vi "AddBatchRuns_DP_ver1.0.vi"(1 "output cluster":T1={"Main Sweep"=0, "Steps Config:"={"total points:"=0, "Step Delay (s)"=0.0, "Ini Delay (s)"=0.0, "# of steps:"=0}, "Temperature Control (ITC 503):"={"GPIB ADR"=0, "Change Heater?"={"Heater?"=FALSE, "Heater"=0}, "Change Temp?"={"Change T?"=FALSE, "Set T (K)"=0.0}, "Cluster"={"Heat Auto?"=FALSE, "Manual Heat?"=FALSE, "Heater (%)"=0.0}, "Change PID?"={"Change PID?"=FALSE, "P"=0.0, "I"=0.0, "D"=0.0}, "Change Para?"=FALSE, "Sensor"=1}, "Temperature Control (LS 340):"={"GPIB ADR"=0, "From (K)"=0.0, "To (K)"=0.0, "Rate (K/min)"=0.0, "Delta T (0.08K)"=0.0, "Temp. Header"="", "T Display Control"={"Ch B"=FALSE, "Ch C"=FALSE, "Ch D"=FALSE}}, "Magnet Control (IPS 120-10)"={"Action"=0, "Standby (s)"=0.0, "Heater on (s)"=0.0, "Sweep Setup "=[], "GPIB ADR"=0, "Change Para?"=FALSE}, "Keithley 6221 :"=[], "Measuring Instruments : "=[], "Lock-In SR7265 :"=[], "Deascription of \nthis measurement"="", "Instruments Config:"=[], "LS372 Bridge : 2"=[{"GPIB"=0, "Excitation"=0, "Autorange?"=FALSE, "Range"=0, "Current"=0, "Voltage"=0, "DataHeader"="Rx;Ry"}], "Magnet Control (CS4) 2"={"Action"=1, "Standby (s)"=0.0, "Heater on (s)"=300.0, "Sweep Setup "=[], "GPIB ADR"=0, "Change Para?"=FALSE}} {"Magnet Control (CS4) 2"."GPIB ADR" items=["None"=0, "25"=25]; "Magnet Control (CS4) 2"."Sweep Setup"."Rate in Range (T/min)" min=0.001 max=0.5 step=0.001; "Magnet Control (CS4) 2"."Sweep Setup"."Hold(min)" min=0.0; "Magnet Control (CS4) 2"."Sweep Setup"."Set Point (T)" min=-9.0 max=9.0 step=0.001; "Magnet Control (CS4) 2"."Action" items=["Up", "Down", "Pause", "Zero"]; "LS372 Bridge : 2"."Voltage" items=["2.00 uV"=1, "6.32 uV"=2, "20.0 uV"=3, "63.2 uV"=4, "200 uV"=5, "632 uV"=6, "2.0 mV"=7, "6.32 mV"=8]; "LS372 Bridge : 2"."Current" items=["1.00 pA"=1, "3.16 pA"=2, "10.0 pA"=3, "31.6 pA"=4, "100 pA"=5, "316 pA"=6, "1.00 nA"=7, "3.16 nA"=8, "10 nA"=9, "31.6 nA"=10, "100 nA"=11, "316 nA"=12, "1.00 uA"=13, "3.16 uA"=14, "10.0 uA"=15, "31.6 uA"=16, "100 uA"=17, "316 uA"=18, "1.00 mA"=19, "3.16 mA"=20, "10.0 mA"=21, "31.6 mA"=22]; "LS372 Bridge : 2"."Range" items=["2.0 m"=1, "6.32 m"=2, "20.0 m"=3, "63.2 m"=4, "200 m"=5, "632 m"=6, "2.00"=7, "6.32"=8, "20.0"=9, "63.2"=10, "200"=11, "632"=12, "2.00 k"=13, "6.32 k"=14, "20.0 k"=15, "63.2 k"=16, "200 k"=17, "632 k"=18, "2.00 M"=19, "6.32 M"=20, "20.0 M"=21, "63.2 M"=22]; "LS372 Bridge : 2"."Excitation" items=["Voltage", "Current"]; "LS372 Bridge : 2"."GPIB" items=["None"=0, "9"=9]; "Main Sweep" items=["Time", "DC Current", "Delta Current", "Pulse Delta Current", "Sine Current", "Lock-in Vosc"]; "Temperature Control (ITC 503):"."Sensor" items=["T2", "T3"]; "Magnet Control (IPS 120-10)"."Action" items=["Hold", "To Set point", "To Zero", "Clamp"]; "Keithley 6221 :"."Sweep Mode" items=["Linear", "Log", "Exp", "Inverse", "Manual"]}) -> (0 "output cluster 2":T1={"Main Sweep"=0, "Steps Config:"={"total points:"=0, "Step Delay (s)"=0.0, "Ini Delay (s)"=0.0, "# of steps:"=0}, "Temperature Control (ITC 503):"={"GPIB ADR"=0, "Change Heater?"={"Heater?"=FALSE, "Heater"=0}, "Change Temp?"={"Change T?"=FALSE, "Set T (K)"=0.0}, "Cluster"={"Heat Auto?"=FALSE, "Manual Heat?"=FALSE, "Heater (%)"=0.0}, "Change PID?"={"Change PID?"=FALSE, "P"=0.0, "I"=0.0, "D"=0.0}, "Change Para?"=FALSE, "Sensor"=1}, "Temperature Control (LS 340):"={"GPIB ADR"=0, "From (K)"=0.0, "To (K)"=0.0, "Rate (K/min)"=0.0, "Delta T (0.08K)"=0.0, "Temp. Header"="", "T Display Control"={"Ch B"=FALSE, "Ch C"=FALSE, "Ch D"=FALSE}}, "Magnet Control (IPS 120-10)"={"Action"=0, "Standby (s)"=0.0, "Heater on (s)"=0.0, "Sweep Setup "=[], "GPIB ADR"=0, "Change Para?"=FALSE}, "Keithley 6221 :"=[], "Measuring Instruments : "=[], "Lock-In SR7265 :"=[], "Deascription of \nthis measurement"="", "Instruments Config:"=[], "LS372 Bridge : 2"=[{"GPIB"=0, "Excitation"=0, "Autorange?"=FALSE, "Range"=0, "Current"=0, "Voltage"=0, "DataHeader"="Rx;Ry"}], "Magnet Control (CS4) 2"={"Action"=1, "Standby (s)"=0.0, "Heater on (s)"=300.0, "Sweep Setup "=[], "GPIB ADR"=0, "Change Para?"=FALSE}} {"Magnet Control (CS4) 2"."GPIB ADR" items=["None"=0, "25"=25]; "Magnet Control (CS4) 2"."Sweep Setup"."Rate in Range (T/min)" min=0.001 max=0.5 step=0.001; "Magnet Control (CS4) 2"."Sweep Setup"."Hold(min)" min=0.0; "Magnet Control (CS4) 2"."Sweep Setup"."Set Point (T)" min=-9.0 max=9.0 step=0.001; "Magnet Control (CS4) 2"."Action" items=["Up", "Down", "Pause", "Zero"]; "LS372 Bridge : 2"."Voltage" items=["2.00 uV"=1, "6.32 uV"=2, "20.0 uV"=3, "63.2 uV"=4, "200 uV"=5, "632 uV"=6, "2.0 mV"=7, "6.32 mV"=8]; "LS372 Bridge : 2"."Current" items=["1.00 pA"=1, "3.16 pA"=2, "10.0 pA"=3, "31.6 pA"=4, "100 pA"=5, "316 pA"=6, "1.00 nA"=7, "3.16 nA"=8, "10 nA"=9, "31.6 nA"=10, "100 nA"=11, "316 nA"=12, "1.00 uA"=13, "3.16 uA"=14, "10.0 uA"=15, "31.6 uA"=16, "100 uA"=17, "316 uA"=18, "1.00 mA"=19, "3.16 mA"=20, "10.0 mA"=21, "31.6 mA"=22]; "LS372 Bridge : 2"."Range" items=["2.0 m"=1, "6.32 m"=2, "20.0 m"=3, "63.2 m"=4, "200 m"=5, "632 m"=6, "2.00"=7, "6.32"=8, "20.0"=9, "63.2"=10, "200"=11, "632"=12, "2.00 k"=13, "6.32 k"=14, "20.0 k"=15, "63.2 k"=16, "200 k"=17, "632 k"=18, "2.00 M"=19, "6.32 M"=20, "20.0 M"=21, "63.2 M"=22]; "LS372 Bridge : 2"."Excitation" items=["Voltage", "Current"]; "LS372 Bridge : 2"."GPIB" items=["None"=0, "9"=9]; "Main Sweep" items=["Time", "DC Current", "Delta Current", "Pulse Delta Current", "Sine Current", "Lock-in Vosc"]; "Temperature Control (ITC 503):"."Sensor" items=["T2", "T3"]; "Magnet Control (IPS 120-10)"."Action" items=["Hold", "To Set point", "To Zero", "Clamp"]; "Keithley 6221 :"."Sweep Mode" items=["Linear", "Log", "Exp", "Inverse", "Manual"]})   [LabVIEW 2012]
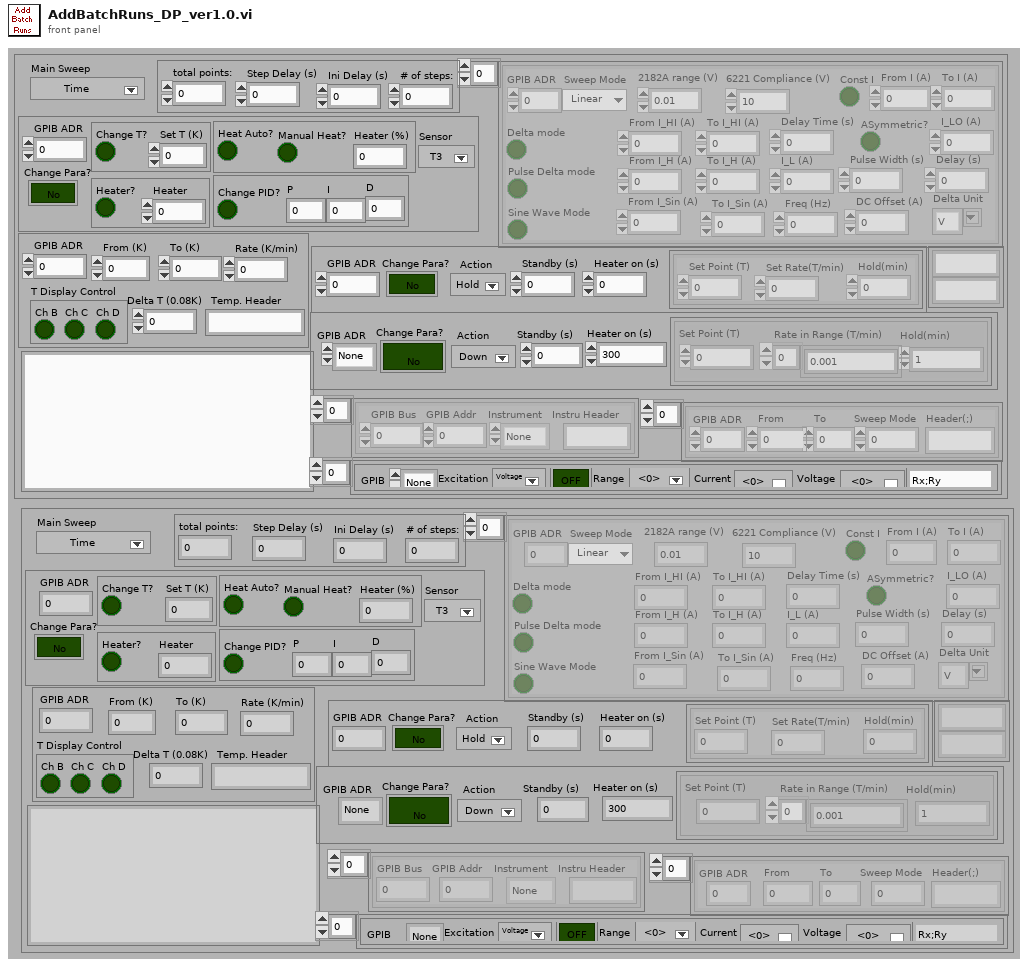
[diagram p1: front panel]
types:
  T1 = cluster{"Main Sweep":u8, "Steps Config:":cluster{"total points:":u32, "Step Delay (s)":dbl, "Ini Delay (s)":dbl, "# of steps:":u32}, "Temperature Control (ITC 503):":cluster{"GPIB ADR":u16, "Change Heater?":cluster{"Heater?":bool, "Heater":u8}, "Change Temp?":cluster{"Change T?":bool, "Set T (K)":dbl}, "Cluster":cluster{"Heat Auto?":bool, "Manual Heat?":bool, "Heater (%)":dbl}, "Change PID?":cluster{"Change PID?":bool, "P":dbl, "I":dbl, "D":dbl}, "Change Para?":bool, "Sensor":u16}, "Temperature Control (LS 340):":cluster{"GPIB ADR":u16, "From (K)":dbl, "To (K)":dbl, "Rate (K/min)":dbl, "Delta T (0.08K)":dbl, "Temp. Header":string, "T Display Control":cluster{"Ch B":bool, "Ch C":bool, "Ch D":bool}}, "Magnet Control (IPS 120-10)":cluster{"Action":u16, "Standby (s)":dbl, "Heater on (s)":dbl, "Sweep Setup ":cluster{"Set Point (T)":dbl, "Set Rate(T/min)":dbl, "Hold(min)":dbl}[], "GPIB ADR":u16, "Change Para?":bool}, "Keithley 6221 :":cluster{"Delta mode":bool, "Const I":bool, "Pulse Delta mode":bool, "Sine Wave Mode":bool, "From I_HI (A)":dbl, "From I (A)":dbl, "I_LO (A)":dbl, "From I_H (A)":dbl, "I_L (A)":dbl, "Freq (Hz)":dbl, "From I_Sin (A)":dbl, "DC Offset (A)":dbl, "Delay Time (s)":dbl, "Pulse Width (s)":dbl, "Delay (s)":dbl, "To I (A)":dbl, "ASymmetric?":bool, "To I_HI (A)":dbl, "To I_H (A)":dbl, "To I_Sin (A)":dbl, "GPIB ADR":u16, "Sweep Mode":u8, "Delta Unit":string, "2182A range (V)":dbl, "6221 Compliance (V)":dbl}[], "Measuring Instruments : ":cluster{"GPIB Bus":dbl, "GPIB Addr":dbl, "Instrument":enum16{"None", "HP34401DMM", "Lockin 7265", "HP3456/7A", "HP3478A", "HP3325FG", "Keithley2182A"}, "Instru Header":string}[], "Lock-In SR7265 :":cluster{"GPIB ADR":u16, "From":dbl, "To":dbl, "Header(;)":string, "Sweep Mode":u8}[], "Deascription of \nthis measurement":string, "Instruments Config:":string[][], "LS372 Bridge : 2":cluster{"GPIB":u16, "Excitation":u16, "Autorange?":bool, "Range":u16, "Current":u16, "Voltage":u16, "DataHeader":string}[], "Magnet Control (CS4) 2":cluster{"Action":u16, "Standby (s)":dbl, "Heater on (s)":dbl, "Sweep Setup ":cluster{"Set Point (T)":dbl, "Hold(min)":dbl, "Rate in Range (T/min)":dbl[]}[], "GPIB ADR":u16, "Change Para?":bool}}
  T2 = cluster{"Delta mode":bool, "Const I":bool, "Pulse Delta mode":bool, "Sine Wave Mode":bool, "From I_HI (A)":dbl, "From I (A)":dbl, "I_LO (A)":dbl, "From I_H (A)":dbl, "I_L (A)":dbl, "Freq (Hz)":dbl, "From I_Sin (A)":dbl, "DC Offset (A)":dbl, "Delay Time (s)":dbl, "Pulse Width (s)":dbl, "Delay (s)":dbl, "To I (A)":dbl, "ASymmetric?":bool, "To I_HI (A)":dbl, "To I_H (A)":dbl, "To I_Sin (A)":dbl, "GPIB ADR":u16, "Sweep Mode":u8, "Delta Unit":string, "2182A range (V)":dbl, "6221 Compliance (V)":dbl}[]
  T3 = cluster{"GPIB ADR":u16, "From":dbl, "To":dbl, "Header(;)":string, "Sweep Mode":u8}[]
  T4 = cluster{"GPIB ADR":u16, "From":dbl, "To":dbl, "Header(;)":string, "Sweep Mode":u8}
  T5 = cluster{"Delta mode":bool, "Const I":bool, "Pulse Delta mode":bool, "Sine Wave Mode":bool, "From I_HI (A)":dbl, "From I (A)":dbl, "I_LO (A)":dbl, "From I_H (A)":dbl, "I_L (A)":dbl, "Freq (Hz)":dbl, "From I_Sin (A)":dbl, "DC Offset (A)":dbl, "Delay Time (s)":dbl, "Pulse Width (s)":dbl, "Delay (s)":dbl, "To I (A)":dbl, "ASymmetric?":bool, "To I_HI (A)":dbl, "To I_H (A)":dbl, "To I_Sin (A)":dbl, "GPIB ADR":u16, "Sweep Mode":u8, "Delta Unit":string, "2182A range (V)":dbl, "6221 Compliance (V)":dbl}
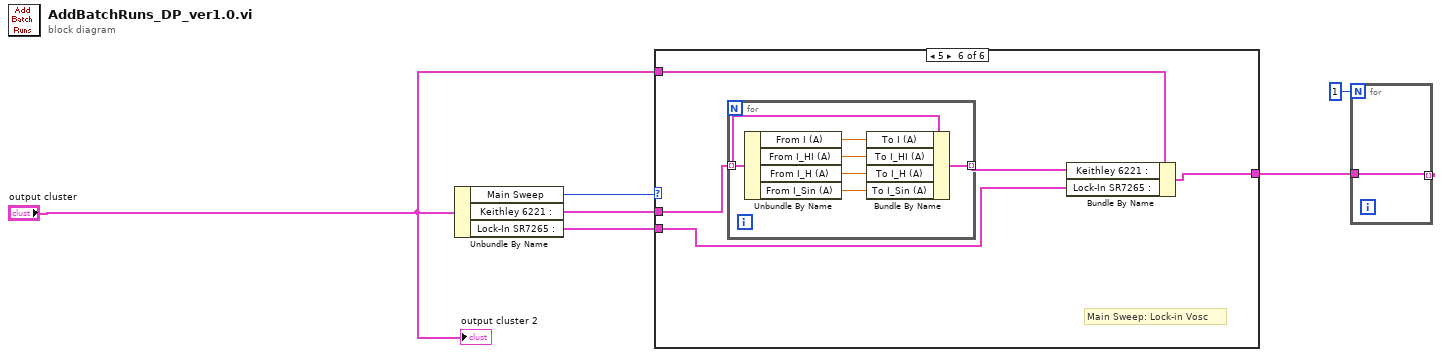
[diagram p0: block diagram]
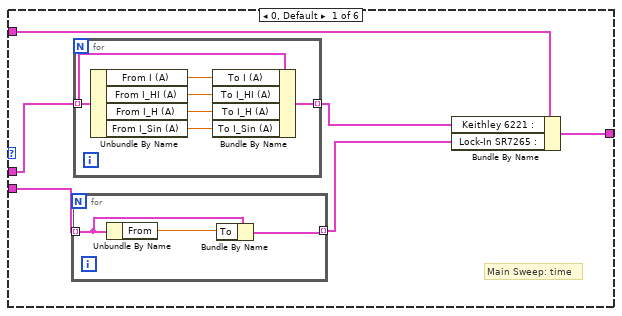
[diagram p2: hidden frame]
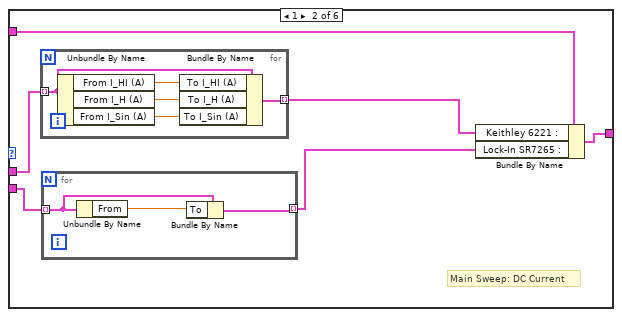
[diagram p3: hidden frame]
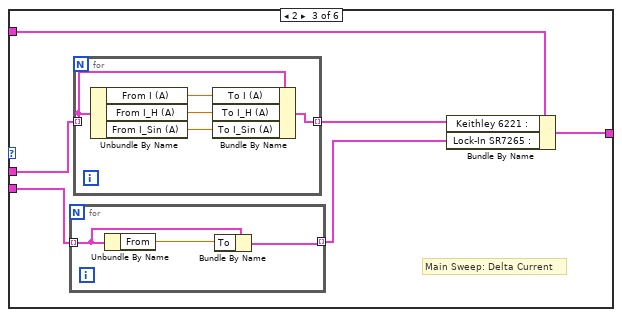
[diagram p4: hidden frame]
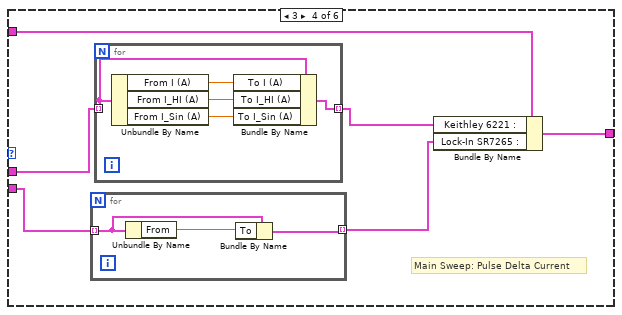
[diagram p5: hidden frame]
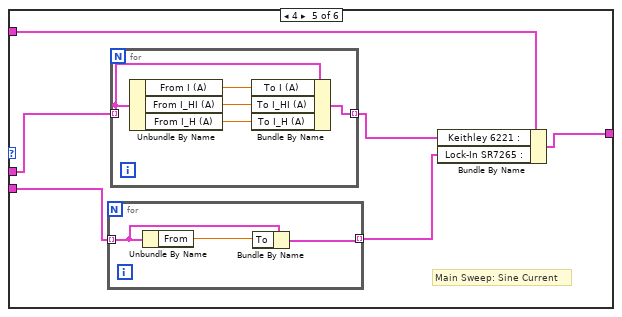
[diagram p6: hidden frame]
diagram:
  n1 = Unbundle By Name("output cluster") -> ("Main Sweep"=w6:u8, "Keithley 6221 :"=w5:T2, "Lock-In SR7265 :"=w4:T3)
  n2 = case shown="5" w6 {
    tunnel: "output cluster" -> [w10 w27 w41 w54 w69 w81]
    tunnel: w5 -> [w12 w25 w39 w53 w67 w80]
    tunnel: w4 -> [w11 w23 w38 w52 w66 w78]
    tunnel: [w7 w26 w40 w55 w68 w82] -> w2
    frame 0, Default {
      # "Main Sweep: time"
      n3 = for {
        tunnel: w11 -> [w15] mode=indexing
        tunnel: [w13] -> w8 mode=indexing
        n4 = Unbundle By Name(w15) -> ("From"=w14:dbl)
        n5 = Bundle By Name(cluster=w15, "To"=w14) -> (w13:T4)
      }
      n6 = for {
        tunnel: w12 -> [w21] mode=indexing
        tunnel: [w17] -> w9 mode=indexing
        n7 = Unbundle By Name(w21) -> ("From I (A)"=w16:dbl, "From I_HI (A)"=w20:dbl, "From I_H (A)"=w19:dbl, "From I_Sin (A)"=w18:dbl)
        n8 = Bundle By Name(cluster=w21, "To I (A)"=w16, "To I_HI (A)"=w20, "To I_H (A)"=w19, "To I_Sin (A)"=w18) -> (w17:T5)
      }
      n9 = Bundle By Name(cluster=w10, "Keithley 6221 :"=w9, "Lock-In SR7265 :"=w8) -> (w7:T1)
    }
    frame 1 {
      # "Main Sweep: DC Current"
      n10 = for {
        tunnel: w25 -> [w35] mode=indexing
        tunnel: [w31] -> w24 mode=indexing
        n11 = Unbundle By Name(w35) -> ("From I_HI (A)"=w34:dbl, "From I_H (A)"=w33:dbl, "From I_Sin (A)"=w32:dbl)
        n12 = Bundle By Name(cluster=w35, "To I_HI (A)"=w34, "To I_H (A)"=w33, "To I_Sin (A)"=w32) -> (w31:T5)
      }
      n13 = for {
        tunnel: w23 -> [w30] mode=indexing
        tunnel: [w28] -> w22 mode=indexing
        n14 = Unbundle By Name(w30) -> ("From"=w29:dbl)
        n15 = Bundle By Name(cluster=w30, "To"=w29) -> (w28:T4)
      }
      n16 = Bundle By Name(cluster=w27, "Keithley 6221 :"=w24, "Lock-In SR7265 :"=w22) -> (w26:T1)
    }
    frame 2 {
      # "Main Sweep: Delta Current"
      n17 = for {
        tunnel: w38 -> [w44] mode=indexing
        tunnel: [w42] -> w36 mode=indexing
        n18 = Unbundle By Name(w44) -> ("From"=w43:dbl)
        n19 = Bundle By Name(cluster=w44, "To"=w43) -> (w42:T4)
      }
      n20 = for {
        tunnel: w39 -> [w49] mode=indexing
        tunnel: [w46] -> w37 mode=indexing
        n21 = Unbundle By Name(w49) -> ("From I (A)"=w45:dbl, "From I_H (A)"=w48:dbl, "From I_Sin (A)"=w47:dbl)
        n22 = Bundle By Name(cluster=w49, "To I (A)"=w45, "To I_H (A)"=w48, "To I_Sin (A)"=w47) -> (w46:T5)
      }
      n23 = Bundle By Name(cluster=w41, "Keithley 6221 :"=w37, "Lock-In SR7265 :"=w36) -> (w40:T1)
    }
    frame 3 {
      # "Main Sweep: Pulse Delta Current"
      n24 = for {
        tunnel: w52 -> [w58] mode=indexing
        tunnel: [w56] -> w50 mode=indexing
        n25 = Unbundle By Name(w58) -> ("From"=w57:dbl)
        n26 = Bundle By Name(cluster=w58, "To"=w57) -> (w56:T4)
      }
      n27 = for {
        tunnel: w53 -> [w63] mode=indexing
        tunnel: [w60] -> w51 mode=indexing
        n28 = Unbundle By Name(w63) -> ("From I (A)"=w59:dbl, "From I_HI (A)"=w62:dbl, "From I_Sin (A)"=w61:dbl)
        n29 = Bundle By Name(cluster=w63, "To I (A)"=w59, "To I_HI (A)"=w62, "To I_Sin (A)"=w61) -> (w60:T5)
      }
      n30 = Bundle By Name(cluster=w54, "Keithley 6221 :"=w51, "Lock-In SR7265 :"=w50) -> (w55:T1)
    }
    frame 4 {
      # "Main Sweep: Sine Current"
      n31 = for {
        tunnel: w66 -> [w72] mode=indexing
        tunnel: [w70] -> w64 mode=indexing
        n32 = Unbundle By Name(w72) -> ("From"=w71:dbl)
        n33 = Bundle By Name(cluster=w72, "To"=w71) -> (w70:T4)
      }
      n34 = for {
        tunnel: w67 -> [w77] mode=indexing
        tunnel: [w74] -> w65 mode=indexing
        n35 = Unbundle By Name(w77) -> ("From I (A)"=w73:dbl, "From I_HI (A)"=w76:dbl, "From I_H (A)"=w75:dbl)
        n36 = Bundle By Name(cluster=w77, "To I (A)"=w73, "To I_HI (A)"=w76, "To I_H (A)"=w75) -> (w74:T5)
      }
      n37 = Bundle By Name(cluster=w69, "Keithley 6221 :"=w65, "Lock-In SR7265 :"=w64) -> (w68:T1)
    }
    frame 5 {
      # "Main Sweep: Lock-in Vosc"
      n38 = for {
        tunnel: w80 -> [w88] mode=indexing
        tunnel: [w84] -> w79 mode=indexing
        n39 = Unbundle By Name(w88) -> ("From I (A)"=w83:dbl, "From I_HI (A)"=w87:dbl, "From I_H (A)"=w86:dbl, "From I_Sin (A)"=w85:dbl)
        n40 = Bundle By Name(cluster=w88, "To I (A)"=w83, "To I_HI (A)"=w87, "To I_H (A)"=w86, "To I_Sin (A)"=w85) -> (w84:T5)
      }
      n41 = Bundle By Name(cluster=w81, "Keithley 6221 :"=w79, "Lock-In SR7265 :"=w78) -> (w82:T1)
    }
  }
  n42 = for {
    N: 1 -> [_]
    tunnel: w2 -> [w89]
    tunnel: [w89] -> _ mode=indexing
  }
  "output cluster 2" <- "output cluster"
